vi "#36_MAV_MSG_SERVO_OUTPUT_RAW.vi"(11 "mavlink_payload":u8[](array[numeric])) -> (3 "SERVO_OUTPUT_RAW":T1)   [LabVIEW 2023]
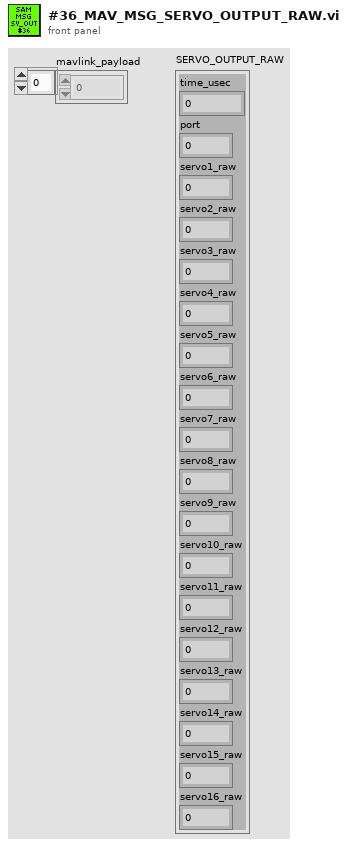
[diagram p1: front panel]
types:
  T1 = cluster{"time_usec":u32, "port":u8, "servo1_raw":u16, "servo2_raw":u16, "servo3_raw":u16, "servo4_raw":u16, "servo5_raw":u16, "servo6_raw":u16, "servo7_raw":u16, "servo8_raw":u16, "servo9_raw":u16, "servo10_raw":u16, "servo11_raw":u16, "servo12_raw":u16, "servo13_raw":u16, "servo14_raw":u16, "servo15_raw":u16, "servo16_raw":u16}
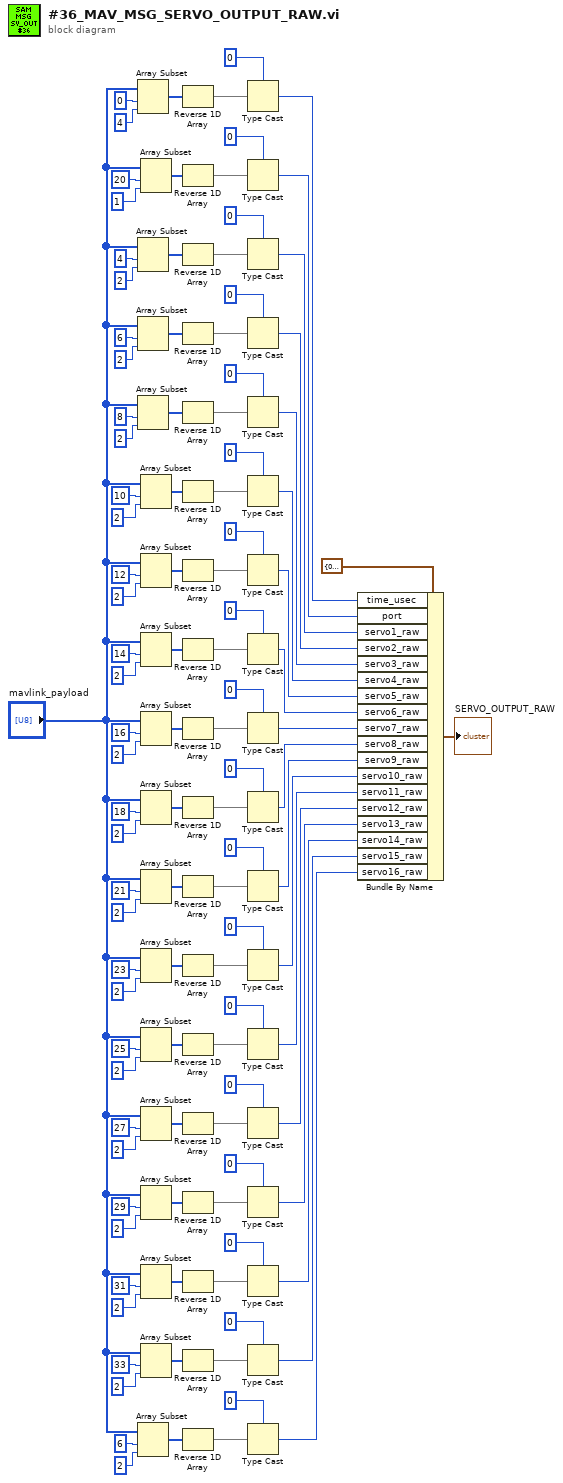
[diagram p0: block diagram]
diagram:
  n1 = Array Subset(array="mavlink_payload", index=0, length=4) -> (w111:u8[])
  n2 = Array Subset(array="mavlink_payload", index=4, length=2) -> (w97:u8[])
  n3 = Array Subset(array="mavlink_payload", index=6, length=2) -> (w91:u8[])
  n4 = Array Subset(array="mavlink_payload", index=8, length=2) -> (w86:u8[])
  n5 = Array Subset(array="mavlink_payload", index=6, length=2) -> (w7:u8[])
  n6 = Array Subset(array="mavlink_payload", index=20, length=1) -> (w103:u8[])
  n7 = Array Subset(array="mavlink_payload", index=10, length=2) -> (w81:u8[])
  n8 = Array Subset(array="mavlink_payload", index=12, length=2) -> (w76:u8[])
  n9 = Array Subset(array="mavlink_payload", index=14, length=2) -> (w67:u8[])
  n10 = Array Subset(array="mavlink_payload", index=16, length=2) -> (w61:u8[])
  n11 = Array Subset(array="mavlink_payload", index=18, length=2) -> (w55:u8[])
  n12 = Array Subset(array="mavlink_payload", index=21, length=2) -> (w49:u8[])
  n13 = Array Subset(array="mavlink_payload", index=23, length=2) -> (w43:u8[])
  n14 = Array Subset(array="mavlink_payload", index=25, length=2) -> (w37:u8[])
  n15 = Array Subset(array="mavlink_payload", index=27, length=2) -> (w31:u8[])
  n16 = Array Subset(array="mavlink_payload", index=29, length=2) -> (w25:u8[])
  n17 = Array Subset(array="mavlink_payload", index=31, length=2) -> (w19:u8[])
  n18 = Array Subset(array="mavlink_payload", index=33, length=2) -> (w13:u8[])
  n19 = Reverse 1D Array(array=w111) -> (reversed array=w110:u8[])
  n20 = Reverse 1D Array(array=w103) -> (reversed array=w102:u8[])
  n21 = Reverse 1D Array(array=w97) -> (reversed array=w96:u8[])
  n22 = Reverse 1D Array(array=w91) -> (reversed array=w90:u8[])
  n23 = Reverse 1D Array(array=w86) -> (reversed array=w85:u8[])
  n24 = Reverse 1D Array(array=w81) -> (reversed array=w80:u8[])
  n25 = Reverse 1D Array(array=w76) -> (reversed array=w75:u8[])
  n26 = Reverse 1D Array(array=w67) -> (reversed array=w66:u8[])
  n27 = Reverse 1D Array(array=w61) -> (reversed array=w60:u8[])
  n28 = Reverse 1D Array(array=w55) -> (reversed array=w54:u8[])
  n29 = Reverse 1D Array(array=w49) -> (reversed array=w48:u8[])
  n30 = Reverse 1D Array(array=w43) -> (reversed array=w42:u8[])
  n31 = Reverse 1D Array(array=w37) -> (reversed array=w36:u8[])
  n32 = Reverse 1D Array(array=w31) -> (reversed array=w30:u8[])
  n33 = Reverse 1D Array(array=w25) -> (reversed array=w24:u8[])
  n34 = Reverse 1D Array(array=w19) -> (reversed array=w18:u8[])
  n35 = Reverse 1D Array(array=w13) -> (reversed array=w12:u8[])
  n36 = Reverse 1D Array(array=w7) -> (reversed array=w6:u8[])
  n37 = Type Cast(type=u32 0 ("index"), x=w110) -> (*(type *) &x=w105:u32)
  n38 = Type Cast(type=u8 0 ("index"), x=w102) -> (*(type *) &x=w98:u8)
  n39 = Type Cast(type=u16 0 ("index"), x=w96) -> (*(type *) &x=w92:u16)
  n40 = Type Cast(type=u16 0 ("index"), x=w90) -> (*(type *) &x=w71:u16)
  n41 = Type Cast(type=u16 0 ("index"), x=w85) -> (*(type *) &x=w70:u16)
  n42 = Type Cast(type=u16 0 ("index"), x=w80) -> (*(type *) &x=w69:u16)
  n43 = Type Cast(type=u16 0 ("index"), x=w75) -> (*(type *) &x=w68:u16)
  n44 = Type Cast(type=u16 0 ("index"), x=w66) -> (*(type *) &x=w62:u16)
  n45 = Type Cast(type=u16 0 ("index"), x=w60) -> (*(type *) &x=w56:u16)
  n46 = Type Cast(type=u16 0 ("index"), x=w54) -> (*(type *) &x=w50:u16)
  n47 = Type Cast(type=u16 0 ("index"), x=w48) -> (*(type *) &x=w44:u16)
  n48 = Type Cast(type=u16 0 ("index"), x=w42) -> (*(type *) &x=w38:u16)
  n49 = Type Cast(type=u16 0 ("index"), x=w36) -> (*(type *) &x=w32:u16)
  n50 = Type Cast(type=u16 0 ("index"), x=w30) -> (*(type *) &x=w26:u16)
  n51 = Type Cast(type=u16 0 ("index"), x=w24) -> (*(type *) &x=w20:u16)
  n52 = Type Cast(type=u16 0 ("index"), x=w18) -> (*(type *) &x=w14:u16)
  n53 = Type Cast(type=u16 0 ("index"), x=w12) -> (*(type *) &x=w8:u16)
  n54 = Type Cast(type=u16 0 ("index"), x=w6) -> (*(type *) &x=w1:u16)
  n55 = Bundle By Name(cluster=T1 {"time_usec"=0, "port"=0, "servo1_raw"=0, "servo2_raw"=0, "servo3_raw"=0, "servo4_raw"=0, "servo5_raw"=0, "servo6_raw"=0, "servo7_raw"=0, "servo8_raw"=0, "servo9_raw"=0, "servo10_raw"=0, "servo11_raw"=0, "servo12_raw"=0, "servo13_raw"=0, "servo14_raw"=0, "servo15_raw"=0, "servo16_raw"=0} ("SERVO_OUTPUT_RAW"), "time_usec"=w105, "port"=w98, "servo1_raw"=w92, "servo2_raw"=w71, "servo3_raw"=w70, "servo4_raw"=w69, "servo5_raw"=w68, "servo6_raw"=w62, "servo7_raw"=w56, "servo8_raw"=w50, "servo9_raw"=w44, "servo10_raw"=w38, "servo11_raw"=w32, "servo12_raw"=w26, "servo13_raw"=w20, "servo14_raw"=w14, "servo15_raw"=w8, "servo16_raw"=w1) -> (→"SERVO_OUTPUT_RAW":T1)
